vi "CalDiaOnlyAll.vi"() -> ()   [LabVIEW 2017]
uses:
  <vilib>/Utility/file.llb/Write To Spreadsheet File (DBL).vi
  <vilib>/Utility/file.llb/Write To Spreadsheet File (string).vi
panel:
  in  "Calibration (1 pixel = ?um)":dbl=1.45
  out "Measurment Progress":u8(slide) scale=0.0..50.0
  out "Quantifying":dbl
  out "Total Video Segments to Quantify":dbl
  # "This VI performs diameter measurements of all videos in the selected folder. The user is prompted to select the folder after which they choose a point on the top vessel wall then a point on the bottom vessel wall. The VI then runs through all the segments and outputs the values into a text file 'Diameter'. Due to dependencies this VI is currently set to use frame 5000 as a template"
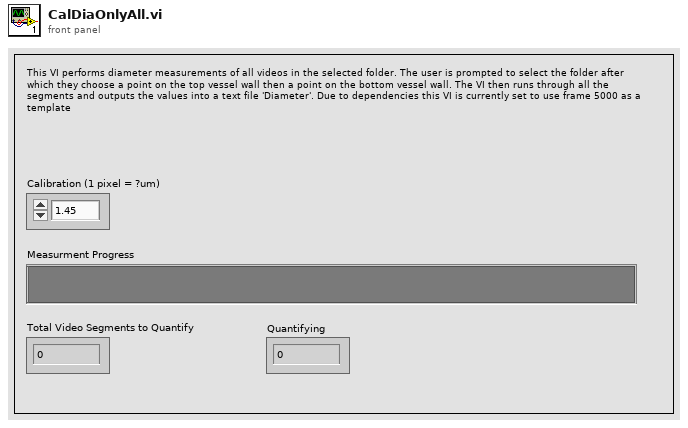
[diagram p1: front panel]
types:
  T1 = typedef "IMAQ AVI2 Refnum.ctl" = refnum<k20>
  T2 = typedef "IMAQ Image.ctl" = refnum<image>
  T3 = typedef "IMAQ Point" = cluster{"X":sgl, "Y":sgl}
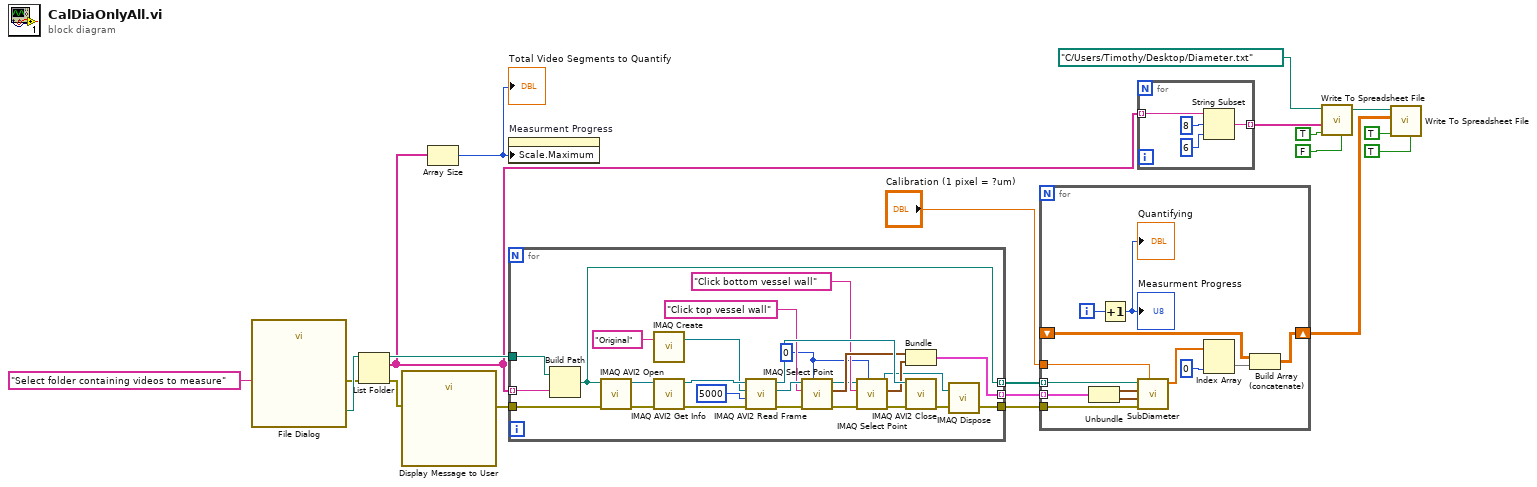
[diagram p0: block diagram]
diagram:
  n1 = call "File Dialog"("prompt"="Select folder containing videos to measure") -> ("selected path"=w19:path, "error out"=w18:errorcluster)  [unwired: 11 in, 2 out]
  n2 = List Folder(path=w19, error in=w18) -> (path out=w16:path, filenames=w5:string[], error out=w12:errorcluster)  [unwired: 2 in, 1 out]
  n3 = call "Display Message to User"("error in (no error)"=w12) -> ("error out"=w11:errorcluster)  [unwired: 9 in, 1 out]
  n4 = Array Size(array=w5) -> (size(s)=w17:i32)
  "Total Video Segments to Quantify" <- w17
  n5 = property on="Measurment Progress" class="Slide (strict)"("Scale.Maximum"=w17) -> ()  [unwired: 2 in, 2 out]
  n6 = for {
    tunnel: w16 -> [w46]
    tunnel: w5 -> [w45] mode=indexing
    tunnel: w11 -> [w37]
    tunnel: [w33] -> w3
    tunnel: [w35] -> w2 mode=indexing
    tunnel: [w25] -> w1 mode=indexing
    w21 = 0 ("Window Number (0...15)")
    n7 = Build Path(base path=w46, name or relative path=w45) -> (appended path=w35:path)
    n8 = call "IMAQ AVI2 Open"("error in (no error)"=w37, "AVI File Path"=w35) -> ("error out"=w43:errorcluster, "AVI Refnum"=w44:T1)  [unwired: 8 in]
    n9 = call "IMAQ Create"("Image Name"="Original") -> ("New Image"=w40:T2)  [unwired: 4 in, 1 out]
    n10 = call "IMAQ AVI2 Get Info"("error in (no error)"=w43, "AVI Refnum"=w44) -> ("error out"=w39:errorcluster, "AVI Refnum (duplicate)"=w42:T1)  [unwired: 5 in, 3 out]
    n11 = call "IMAQ AVI2 Read Frame"("error in (no error)"=w39, "Frame Number"=u32 5000, "Image"=w40, "AVI Refnum"=w42) -> ("error out"=w32:errorcluster, "Image Out"=w31:T2, "AVI Refnum (duplicate)"=w36:T1)  [unwired: 5 in]
    n12 = call "IMAQ Select Point"("Window Number (0...15)"=w21, "error in (no error)"=w32, "Prompt"="Click top vessel wall", "Image In"=w31) -> ("error out"=w29:errorcluster, "Point"=w26:T3, "Image Out (duplicate)"=w22:T2)  [unwired: 4 in, 1 out]
    n13 = call "IMAQ Select Point"("Window Number (0...15)"=w21, "error in (no error)"=w29, "Prompt"="Click bottom vessel wall", "Image In"=w22) -> ("error out"=w28:errorcluster, "Point"=w27:T3, "Image Out (duplicate)"=w23:T2)  [unwired: 4 in, 1 out]
    n14 = Bundle("Point"=w26, "Point"=w27) -> (w25:cluster{"Point":T3, "Point":T3})  [unwired: 1 in]
    n15 = call "IMAQ AVI2 Close"("error in (no error)"=w28, "AVI Refnum"=w36) -> ("error out"=w34:errorcluster)  [unwired: 9 in]
    n16 = call "IMAQ Dispose"("Image"=w23, "error in (no error)"=w34) -> ("error out"=w33:errorcluster)  [unwired: 4 in]
  }
  n17 = for {
    tunnel: w3 -> [w59]
    tunnel: w2 -> [w52] mode=indexing
    tunnel: "Calibration (1 pixel = ?um)" -> [w51]
    shift-right: [w58] -> w13
    shift-left: _ -> [w57]
    tunnel: w1 -> [w49] mode=indexing
    i -> [w54]
    n18 = Unbundle(w49) -> ("Point"=w48:T3, "Point"=w47:T3)
    n19 = Increment(x=w54) -> (x+1=→"Quantifying" →"Measurment Progress":i32)
    n20 = call "SubDiameter.vi"("Calibration (1 pixel = ?um)"=w51, "error in (no error)"=w59, "Bot Wall"=w47, "Top wall"=w48, "AVI Path"=w52) -> ("Diameter"=w50:dbl[])  [unwired: 3 in, 3 out]
    n21 = Index Array(array=w50, index (col)=0 ("index (row)")) -> (element=w56:dbl[])  [unwired: 1 in]
    n22 = Build Array (concatenate)(w57, w56) -> (w58:dbl[][])
  }
  n23 = for {
    tunnel: w5 -> [w63] mode=indexing
    tunnel: [w60] -> w4 mode=indexing
    n24 = String Subset(string=w63, offset (0)=8, length (rest)=6 ("length (rest)")) -> (substring=w60:string)
  }
  n25 = call-poly <vilib>:"Write To Spreadsheet File.vi"("transpose? (no:F)"=FALSE, "append to file? (new file:F)"=TRUE, "1D data"=w4, "file path (dialog if empty)"=path "C:/Users/Timothy/Desktop/Diameter.txt") -> ("new file path (Not A Path if cancelled)"=w7:path)  [unwired: 4 in]
  n26 = call-poly <vilib>:"Write To Spreadsheet File.vi"("transpose? (no:F)"=TRUE, "append to file? (new file:F)"=TRUE, "2D data"=w13, "file path (dialog if empty)"=w7) -> ()  [unwired: 4 in, 1 out]
